vi "空泡图像叠加.vi"(9 "Image Src A":T1, 11 "Image Src":T1) -> (3 "Image Dst Out":T1)   [LabVIEW 2018]
uses:
  <vilib>/vision/Image Controls.llb/IMAQ Image.ctl
  <vilib>/Utility/error.llb/DialogType.ctl
  <vilib>/vision/NI_Vision_Development_Module.lvlib
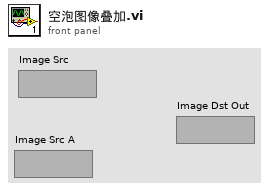
[diagram p1: front panel]
types:
  T1 = typedef "IMAQ Image.ctl" = refnum<image>
  T2 = typedef "DialogType.ctl" = u16
  T3 = typedef "Image Type" = u32
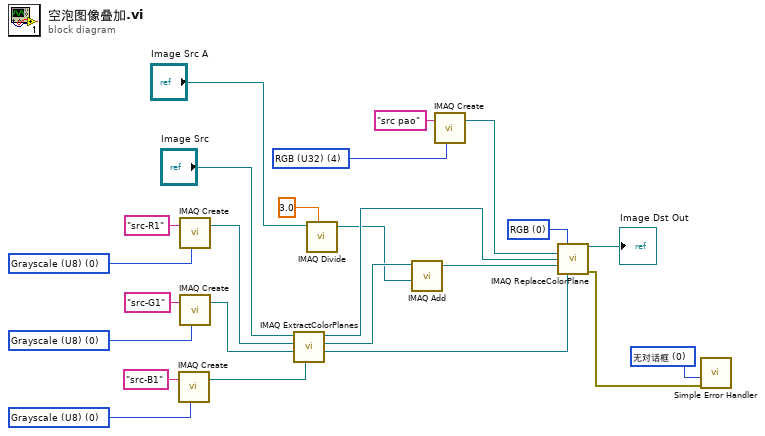
[diagram p0: block diagram]
diagram:
  w2 = T2 0 items=["无对话框", "确定信息", "继续或停止信息", "确定信息＋警告", "继续/停止+警告"] ("type of dialog (OK msg:1)")
  w12 = T3 4 items=["Grayscale (U8)", "Grayscale (I16)", "Grayscale (SGL)", "Complex (CSG)", "RGB (U32)", "HSL (U32)", "RGB (U64)", "Grayscale (U16)"] ("Image Type")
  w14 = u16 0 items=["RGB", "HSL", "HSV", "HSI"] ("Color Mode")
  w19 = T3 0 items=["Grayscale (U8)", "Grayscale (I16)", "Grayscale (SGL)", "Complex (CSG)", "RGB (U32)", "HSL (U32)", "RGB (U64)", "Grayscale (U16)"] ("Image Type")
  w20 = T3 0 items=["Grayscale (U8)", "Grayscale (I16)", "Grayscale (SGL)", "Complex (CSG)", "RGB (U32)", "HSL (U32)", "RGB (U64)", "Grayscale (U16)"] ("Image Type")
  w21 = T3 0 items=["Grayscale (U8)", "Grayscale (I16)", "Grayscale (SGL)", "Complex (CSG)", "RGB (U32)", "HSL (U32)", "RGB (U64)", "Grayscale (U16)"] ("Image Type")
  n1 = call "IMAQ Create"("Image Name"="src-B1", "Image Type"=w19) -> ("New Image"=w15:T1)  [unwired: 3 in, 1 out]
  n2 = call "IMAQ Create"("Image Name"="src-R1", "Image Type"=w21) -> ("New Image"=w18:T1)  [unwired: 3 in, 1 out]
  n3 = call "IMAQ Create"("Image Name"="src-G1", "Image Type"=w20) -> ("New Image"=w17:T1)  [unwired: 3 in, 1 out]
  n4 = call "IMAQ ExtractColorPlanes"("Blue or Luma or Val or Inten Plane"=w15, "Green or Sat Plane"=w17, "Red or Hue Plane"=w18, "Image Src"="Image Src") -> ("Blue or Luma or Val or Inten Plane out"=w9:T1, "Green or Sat Plane out"=w10:T1, "Red or Hue Plane out"=w16:T1)  [unwired: 4 in, 1 out]
  n5 = call "IMAQ Divide"("Image Src A"="Image Src A", "Constant"=3.0) -> ("Image Dst Out"=w7:T1)  [unwired: 5 in, 1 out]
  n6 = call "IMAQ Add"("Image Src A"=w10, "Image Src B"=w7) -> ("Image Dst Out"=w6:T1)  [unwired: 5 in, 1 out]
  n7 = call "IMAQ Create"("Image Name"="src pao", "Image Type"=w12) -> ("New Image"=w11:T1)  [unwired: 3 in, 1 out]
  n8 = call "IMAQ ReplaceColorPlane"("Color Mode"=w14, "Image Dst"=w11, "Red or Hue Plane"=w16, "Green or Sat Plane"=w6, "Blue or Luma or Val or Inten Plane"=w9) -> ("Image Dst Out"=→"Image Dst Out":T1, "error out"=w1:errorcluster)  [unwired: 9 in]
  n9 = call <vilib>:"Simple Error Handler.vi"("type of dialog (OK msg:1)"=w2, "error in (no error)"=w1) -> ()  [unwired: 3 in, 5 out]
